vi "Read 2400 Data (SubVI).vi"(11 "簇":T1 {"Instrument"."Input (0:A)" items=["A", "B"]; "Instrument"."Instrument Type" items=["PPMS", "VersaLab", "DynaCool", "SVSM", "Lakeshore335", "PPMS-Rotate"]; "Instrument"."Heater Output (1:1)" items=["1"=1, "2"=2]; "SR830+6221"."source" items=["SR830 1", "SR830 2", "SR830 3", "SR830 4"]}) -> (3 "数组":string[](array[string]))   [LabVIEW 2019, in "SubVI.lvlib"]
uses:
  SubVI.lvlib
  config.ctl
  <vilib>/NI/Modbus Library/API/Master/Modbus Master.lvclass
  Instrument.ctl
  lib/QDInstrument.dll
  lib/Keithley 24XX/Public/Data/Read (Single Point).vi
  lib/Keithley 24XX/Keithley 24XX.lvlib
panel:
  # "(真是通道1，假是通道2)"
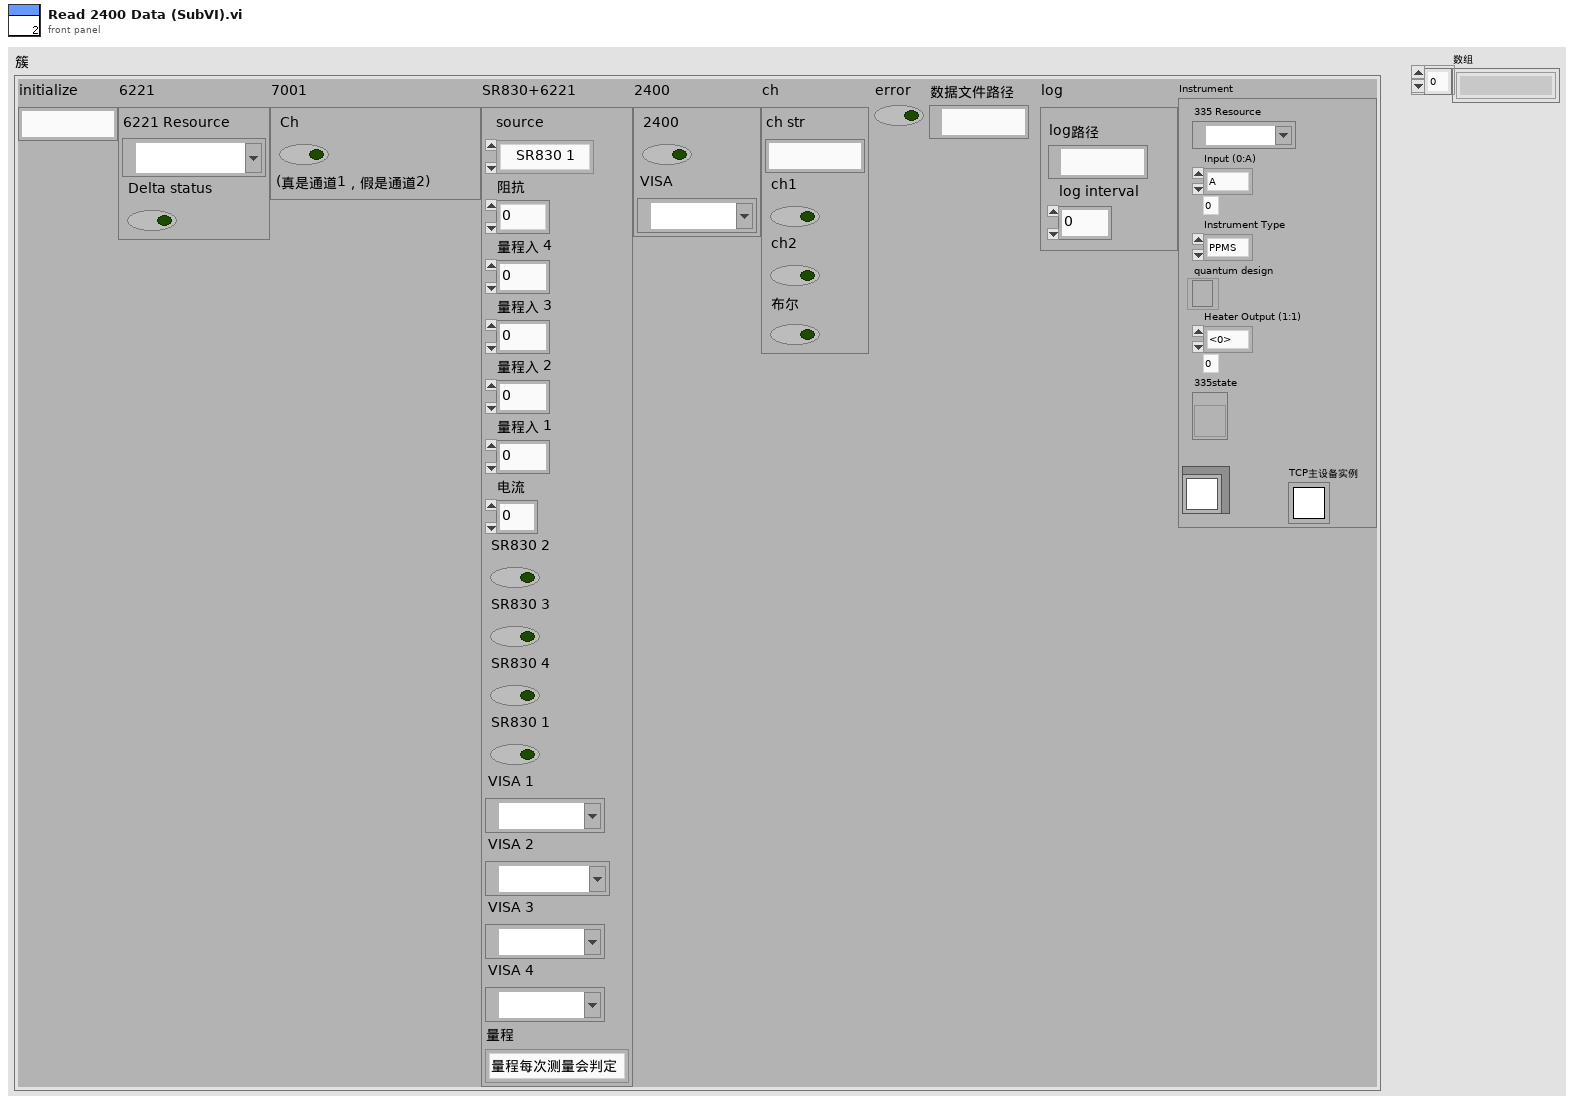
[diagram p1: front panel]
types:
  T1 = typedef "config.ctl" = cluster{"initialize":string, "6221":cluster{"6221 Resource":refnum<visa-resource-name>, "Delta status":bool}, "7001":cluster{"Ch":bool}, "SR830+6221":cluster{"source":u16, "阻抗":dbl, "量程入 4":i32, "量程入 3":i32, "量程入 2":i32, "量程入 1":i32, "电流":dbl, "SR830 2":bool, "SR830 3":bool, "SR830 4":bool, "SR830 1":bool, "VISA 1":refnum<visa-resource-name>, "VISA 2":refnum<visa-resource-name>, "VISA 3":refnum<visa-resource-name>, "VISA 4":refnum<visa-resource-name>, "量程":enum16{"量程每次测量会判定", "量程不变为设定值"}}, "2400":cluster{"2400":bool, "VISA":refnum<visa-resource-name>}, "ch":cluster{"ch str":string, "ch1":bool, "ch2":bool, "布尔":bool}, "error":bool, "数据文件路径":path, "log":cluster{"log路径":path, "log interval":dbl}, "Instrument":T2}
  T2 = typedef "Instrument.ctl" = cluster{"335 Resource":refnum<visa-resource-name>, "Input (0:A)":u16, "Instrument Type":i32, "quantum design":refnum<k24>, "Heater Output (1:1)":u16, "335state":refnum<vi>, "semaphore":T3, "TCP master instance":refnum<class "Modbus Master.lvclass">}
  T3 = typedef "Semaphore RefNum" = refnum<k1>
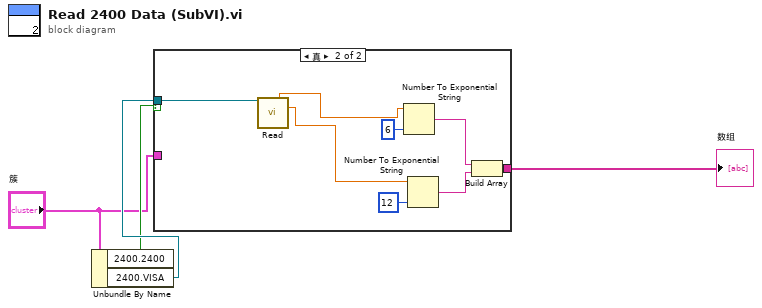
[diagram p0: block diagram]
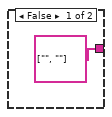
[diagram p2: hidden frame]
diagram:
  n1 = Unbundle By Name("簇") -> ("2400.2400"=w2:bool, "2400.VISA"=w3:refnum<visa-resource-name>)
  n2 = case shown="真" w2 {
    tunnel: w3 -> [_ w13]
    tunnel: [string[] ["", ""] w6] -> w4
    tunnel: "簇" -> [_ _]
    frame False {
    }
    frame True {
      n3 = call-poly "Read.vi"("VISA resource name"=w13) -> ("Voltage"=w12:sgl, "Current"=w10:sgl)  [unwired: 8 in, 5 out]
      n4 = Number To Exponential String(number=w12, precision (6)=i16 6 ("精度(6)")) -> (E-format string=w8:string)  [unwired: 2 in]
      n5 = Number To Exponential String(number=w10, precision (6)=i16 12 ("精度(6)")) -> (E-format string=w7:string)  [unwired: 2 in]
      n6 = Build Array(w8, w7) -> (w6:string[])
    }
  }
  "数组" <- w4
